vi "Set Producer Values.vi"(8 "error in":errorcluster, 9 "Producer Ch":T1[](array[typedef]), 10 "Producer Control":T2, 11 "Climate Chamber Cluster.lvclass in":refnum<class "Climate Chamber Cluster.lvclass">) -> (0 "error out":errorcluster, 3 "Climate Chamber Cluster.lvclass out":refnum<class "Climate Chamber Cluster.lvclass">)   [LabVIEW 2023, in "Climate Chamber Cluster.lvclass"]
uses:
  Climate Chamber Cluster.lvclass
  Producer Control.ctl
  Producer Ch.ctl
  Climate Chamber Cluster.lvclass/Climate Chamber Cluster.ctl
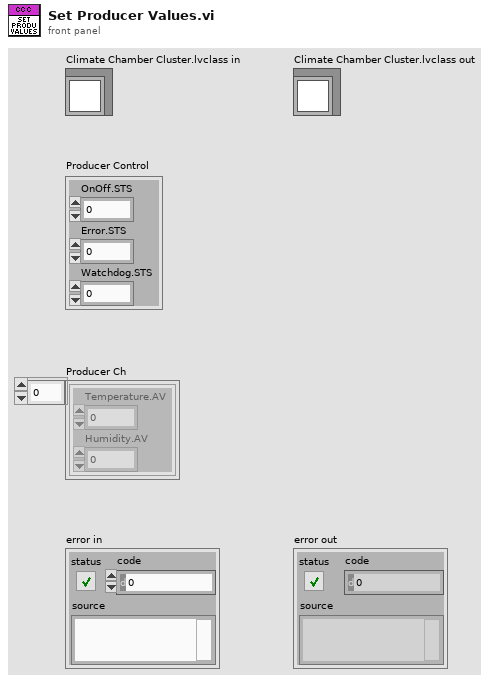
[diagram p1: front panel]
types:
  T1 = typedef "Climate Chamber Cluster.lvclass/Producer Ch.ctl" = cluster{"Temperature.AV":dbl, "Humidity.AV":dbl}
  T2 = typedef "Climate Chamber Cluster.lvclass/Producer Control.ctl" = cluster{"OnOff.STS":i32, "Error.STS":i32, "Watchdog.STS":i32}
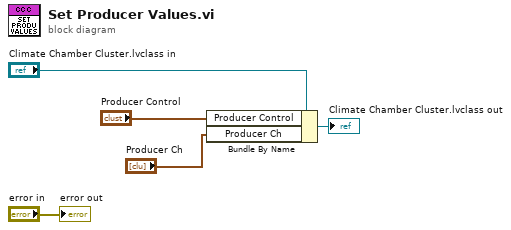
[diagram p0: block diagram]
diagram:
  n1 = Bundle By Name(cluster="Climate Chamber Cluster.lvclass in", "Producer Control"="Producer Control", "Producer Ch"="Producer Ch") -> (→"Climate Chamber Cluster.lvclass out":refnum<class "Climate Chamber Cluster.lvclass">)
  "error out" <- "error in"
